vi "op_biti_v1.vi"() -> ()   [LabVIEW 2009]
panel:
  out "Numeric 8":dbl
  out "Numeric 7":dbl
  out "Numeric 6":dbl
  out "Numeric 5":dbl
  out "Numeric 4":dbl=1.0
  out "Numeric 3":dbl
  out "Numeric 2":dbl=1.0
  out "Numeric1":dbl
  out "Boolean 8":bool
  out "Boolean 7":bool
  out "Boolean 6":bool
  out "Boolean 5":bool
  out "Boolean 4":bool=TRUE
  out "Boolean 3":bool
  out "Boolean 2":bool=TRUE
  out "Boolean1":bool
  in  "Numeric 9":u8=10
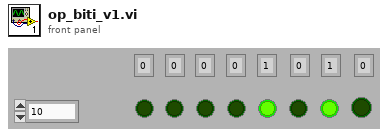
[diagram p1: front panel]
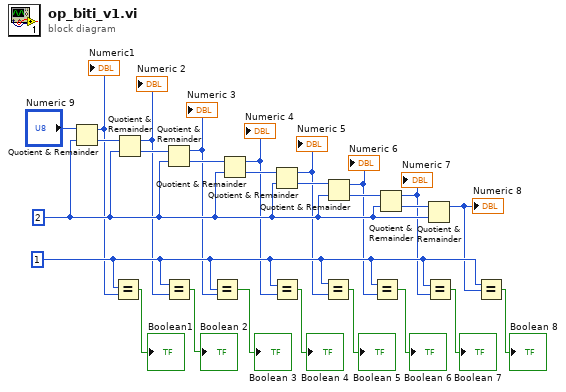
[diagram p0: block diagram]
diagram:
  w8 = 2
  w20 = 1
  n1 = Quotient & Remainder(x="Numeric 9", y=w8) -> (x-y*floor(x/y)=w1:i32, floor(x/y)=w11:i32)
  "Numeric1" <- w1
  n2 = Equal?(x=w20, y=w1) -> (x = y?=→"Boolean1":bool)
  n3 = Quotient & Remainder(x=w11, y=w8) -> (x-y*floor(x/y)=w2:i32, floor(x/y)=w10:i32)
  "Numeric 2" <- w2
  n4 = Quotient & Remainder(x=w10, y=w8) -> (x-y*floor(x/y)=w3:i32, floor(x/y)=w9:i32)
  "Numeric 3" <- w3
  n5 = Equal?(x=w20, y=w2) -> (x = y?=→"Boolean 2":bool)
  n6 = Equal?(x=w20, y=w3) -> (x = y?=→"Boolean 3":bool)
  n7 = Quotient & Remainder(x=w9, y=w8) -> (x-y*floor(x/y)=w4:i32, floor(x/y)=w12:i32)
  "Numeric 4" <- w4
  n8 = Quotient & Remainder(x=w12, y=w8) -> (x-y*floor(x/y)=w5:i32, floor(x/y)=w13:i32)
  "Numeric 5" <- w5
  n9 = Equal?(x=w20, y=w4) -> (x = y?=→"Boolean 4":bool)
  n10 = Equal?(x=w20, y=w5) -> (x = y?=→"Boolean 5":bool)
  n11 = Quotient & Remainder(x=w13, y=w8) -> (x-y*floor(x/y)=w6:i32, floor(x/y)=w14:i32)
  "Numeric 6" <- w6
  n12 = Equal?(x=w20, y=w6) -> (x = y?=→"Boolean 6":bool)
  n13 = Quotient & Remainder(x=w14, y=w8) -> (x-y*floor(x/y)=w7:i32, floor(x/y)=w15:i32)
  "Numeric 7" <- w7
  n14 = Quotient & Remainder(x=w15, y=w8) -> (x-y*floor(x/y)=w19:i32)  [unwired: 1 out]
  "Numeric 8" <- w19
  n15 = Equal?(x=w20, y=w7) -> (x = y?=→"Boolean 7":bool)
  n16 = Equal?(x=w20, y=w19) -> (x = y?=→"Boolean 8":bool)
